vi "Byte Buffer.Subset.vi"(8 "error in (no error)":errorcluster, 9 "length":i32, 10 "buffer offset (0)":i32, 11 "buffer in":string) -> (0 "error out":errorcluster, 2 "buffer subset":string, 3 "buffer out":string)   [LabVIEW 2016, in "VeriStand Data.lvlib"]
uses:
  VeriStand Data.lvlib
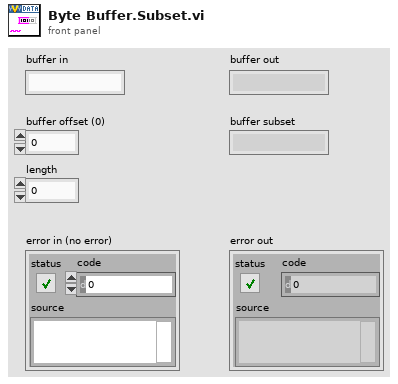
[diagram p1: front panel]
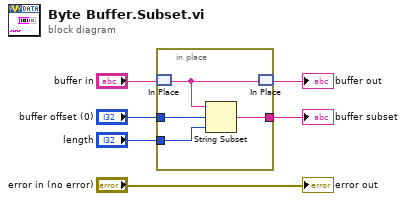
[diagram p0: block diagram]
diagram:
  n1 = in-place {
    in-place-border: "buffer offset (0)" -> [w9]
    in-place-border: "length" -> [w8]
    in-place-border: [w7] -> w2
    n2 = in-place-match #1("buffer in") -> (w10:string)
    n3 = String Subset(string=w10, offset (0)=w9, length (rest)=w8) -> (substring=w7:string)
    n4 = in-place-match #1(w10) -> (→"buffer out":string)
  }
  "buffer subset" <- w2
  "error out" <- "error in (no error)"
